vi "Z6_Beamline.set 6P Switch State in GUI.vi"(0 "i ref in":refnum<vi>, 2 "6P Switch  Name":string="N/A", 3 "Status":T1 items=["no info", "off/false/out", "on/true/in", "Failure", "Alarm", "Status 1", "Status 2", "Status 3"], 4 "No link? (false)":bool, 5 "error in":errorcluster) -> (14 "i ref out":refnum<vi>, 19 "error out":errorcluster)   [LabVIEW 2009]
doc: "This VI sets the 6P Switch State GUI object."
uses:
  Z6_Beamline.lvlib
  PH_Common/Ctrls/Shutter State.ctl
  CSUser/DIMServiceTools/Status.ctl
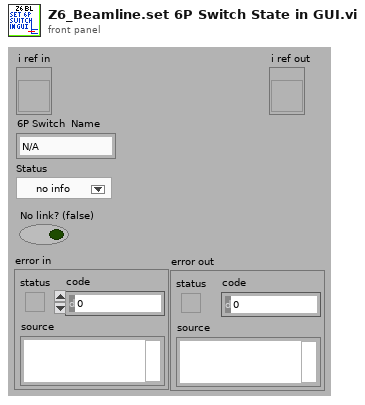
[diagram p1: front panel]
types:
  T1 = typedef "Status.ctl" = i16
  T2 = typedef "Shutter State.ctl" = enum16{"No Link", "No Info", "In", "Out", "in between"}
  T3 = typedef "Z6_Beamline.lvlib/Z6_Beamline.i attribute.ctl" = cluster{"GUI Refs":cluster{"Northtower ok":refnum<vi>, "Southtower ok":refnum<vi>, "Frontends ok":refnum<vi>, "100TW COS ok":refnum<vi>}, "Refs BL Northtower":refnum<vi>[], "Refs BL Southtower":refnum<vi>[], "Refs BL 100TW COS":refnum<vi>[], "Color State PHELIX":cluster{"Service Name":string, "State":i16}, "State Subsystems":cluster{"Northtower":bool, "Southtower":bool, "Frontends":bool, "100TW COS":bool}}
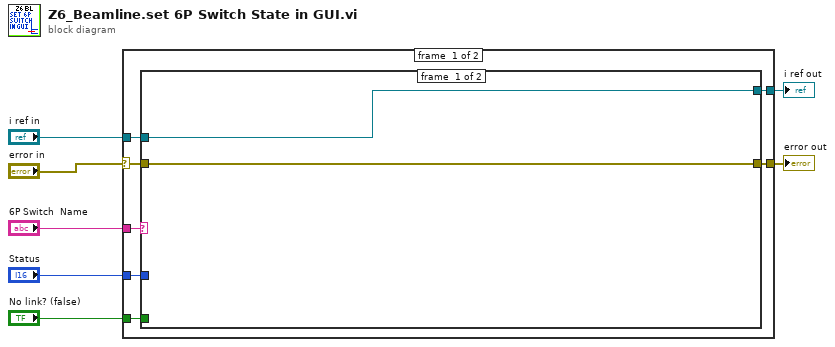
[diagram p0: block diagram]
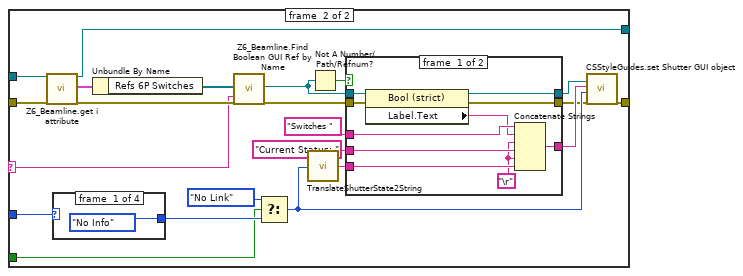
[diagram p2: hidden frame]
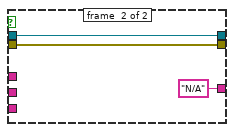
[diagram p3: hidden frame]
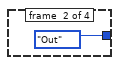
[diagram p4: hidden frame]
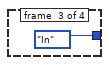
[diagram p5: hidden frame]
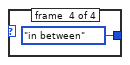
[diagram p6: hidden frame]
diagram:
  n1 = case shown="No Error" "error in" {
    selector: "error in" -> [w8 w57]
    tunnel: "Status" -> [w14 _]
    tunnel: [w13 w57] -> w6
    tunnel: [w12 w56] -> w5
    tunnel: "i ref in" -> [w11 w56]
    tunnel: "No link? (false)" -> [w10 _]
    tunnel: "6P Switch  Name" -> [w9 _]
    frame #0 {
      n2 = case shown="Default" w9 {
        selector: w9 -> [_ w27]
        tunnel: w14 -> [_ w38]
        tunnel: [w15 w37] -> w13
        tunnel: [w16 w35] -> w12
        tunnel: w11 -> [w16 w32]
        tunnel: w8 -> [w15 w31]
        tunnel: w10 -> [_ w28]
        frame #0 {
        }
        frame #1 {
          n3 = call "Z6_Beamline.get i attribute.vi"("i ref in"=w32, "error in (no error)"=w31) -> ("i ref out"=w35:refnum<vi>, "i attribute"=w33:T3, "error out"=w36:errorcluster)  [unwired: 15 in]
          n4 = case shown="5" w38 {
            tunnel: [Shutter_State."No Info" ("Shutter State") Shutter_State."Out" ("Shutter State") Shutter_State."In" ("Shutter State") Shutter_State."in between" ("Shutter State")] -> w30
            frame #0 {
            }
            frame #1 {
            }
            frame #2 {
            }
            frame #3 {
            }
          }
          n5 = Unbundle By Name(w33) -> ("Refs 6P Switches"=w34:refnum<vi>[])
          n6 = call "Z6_Beamline.Find Boolean GUI Ref by Name.vi"("Ref Array"=w34, "Label"=w27, "error in (no error)"=w36) -> ("Wanted Ref"=w22:refnum<vi>, "error out"=w21:errorcluster)  [unwired: 13 in, 2 out]
          n7 = Select(t=Shutter_State."No Link" ("Shutter State"), s=w28, f=w30) -> (s? t:f=w20:T2)
          n8 = call "TranslateShutterState2String.vi"("Shutter State"=w20) -> ("String"=w23:string)
          n9 = Not A Number/Path/Refnum?(number/path/refnum=w22) -> (NaN/Path/Refnum?=w26:bool)
          n10 = case shown="False" w26 {
            tunnel: "Current Status: " ("string") -> [w48 _]
            tunnel: w23 -> [w47 _]
            tunnel: [w41 w51] -> w17
            tunnel: "Switches " ("string") -> [w46 _]
            tunnel: w21 -> [w45 w51]
            tunnel: w22 -> [w44 w50]
            tunnel: [w40 w50] -> w18
            tunnel: [w39 "N/A"] -> w19
            frame #0 {
              w42 = "\r"
              n11 = property class="Bool (strict)"(reference=w44, error in=w45) -> (reference out=w40:refnum<vi>, error out=w41:errorcluster, "Label.Text"=w43:string)
              n12 = Concatenate Strings(w46, w43, w42, w48, w42, w47) -> (w39:string)
            }
            frame #1 {
            }
          }
          n13 = call "CSStyleGuides.set Shutter GUI object.vi"("Ref Object"=w18, "Tip Strip"=w19, "Shutter State"=w20, "error in (no error)"=w17) -> ("error out"=w37:errorcluster)  [unwired: 15 in]
        }
      }
    }
    frame #1 {
    }
  }
  "error out" <- w6
  "i ref out" <- w5
